vi "Set Intensity Graph Z Color.vi"(8 "error in (no error)":errorcluster, 10 "Colors []":u32[](array[colorbox])=[10420479, 16860, 3381759, 6618880, 16772608, 16711680], 11 "graph_utilities in":refnum<class "graph_utilities.lvclass">) -> (0 "error out":errorcluster, 3 "graph_utilities out":refnum<class "graph_utilities.lvclass">)   [LabVIEW 2016, in "graph_utilities.lvclass"]
doc: "Define a Z Scale color table for the Intensity Graph. Default colors are rainbow."
uses:
  graph_utilities.lvclass
  graph_utilities.lvclass/graph_utilities.ctl
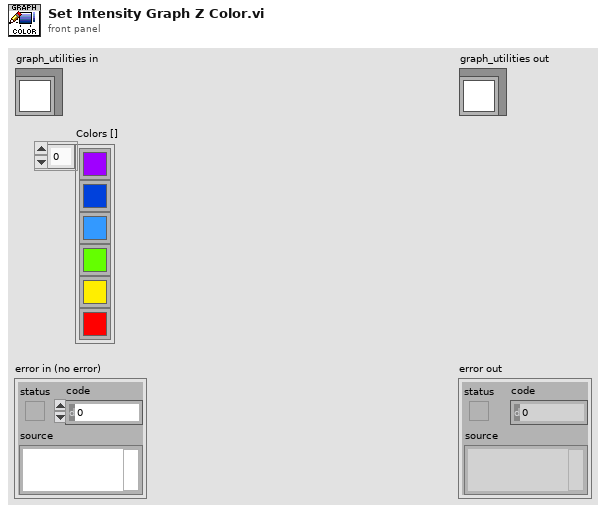
[diagram p1: front panel]
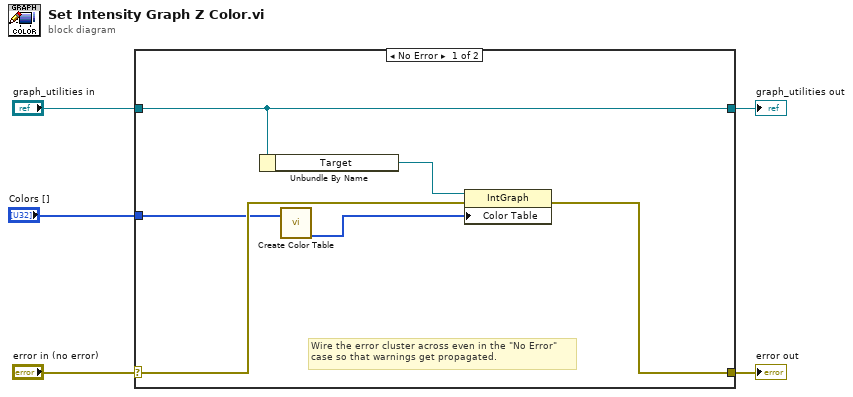
[diagram p0: block diagram]
diagram:
  n1 = case shown="No Error" "error in (no error)" {
    selector: "error in (no error)" -> [w9 w13]
    tunnel: [w8 w13] -> w4
    tunnel: [w11 w12] -> w2
    tunnel: "graph_utilities in" -> [w11 w12]
    tunnel: "Colors []" -> [w7 _]
    frame No Error {
      # "Wire the error cluster across even in the \"No Error\"\ncase so that warnings get propagated."
      n2 = Unbundle By Name(w11) -> ("Target"=w10:refnum<vi>)
      n3 = call "Create Color Table.vi"("Colors []"=w7) -> ("Color Tbl"=w6:u32[])  [unwired: 1 in, 3 out]
      n4 = property on="Property Node" class="IntGraph"(reference=w10, error in=w9, "Color Table"=w6) -> (error out=w8:errorcluster)  [unwired: 1 out]
    }
    frame Error {
    }
  }
  "error out" <- w4
  "graph_utilities out" <- w2
